vi "Read Tektronix Configuration.vi"(8 "error in (no error)":errorcluster, 11 "Tektronix Driver in":refnum<class "Tektronix Driver.lvclass">) -> (0 "error out":errorcluster, 2 "Tektronix Configuration":T1={"Channel"=0, "Number of averages"=4096, "Input Impedance"=0, "Timebase"=1e-06, "Input range"=2.0} {"Input range" format="%#_6pV"; "Timebase" format="%#_6ps"; "Input Impedance" items=["1M", "50", "Isolated"]}, 3 "Tektronix Driver out":refnum<class "Tektronix Driver.lvclass">)   [LabVIEW 2021, in "Tektronix Driver.lvclass"]
uses:
  Tektronix Driver.lvclass
  Tektronix Configuration.ctl
  Tektronix Driver.lvclass/Tektronix Driver.ctl
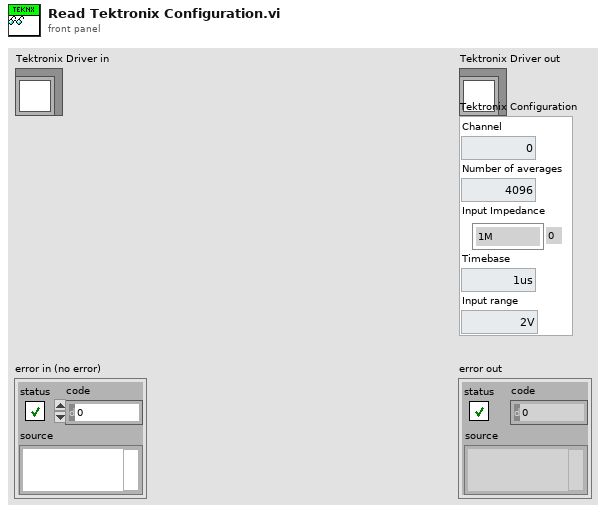
[diagram p1: front panel]
types:
  T1 = typedef "Tektronix Configuration.ctl" = cluster{"Channel":i32, "Number of averages":i32, "Input Impedance":u16, "Timebase":dbl, "Input range":dbl}
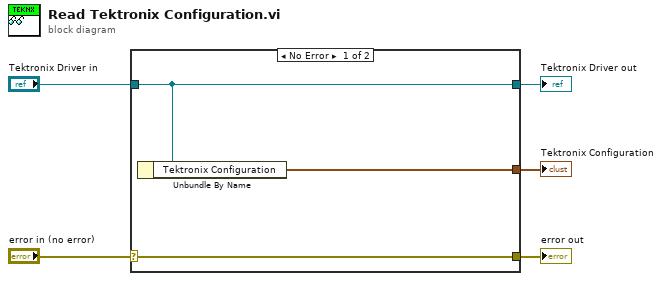
[diagram p0: block diagram]
diagram:
  n1 = case shown="No Error" "error in (no error)" {
    selector: "error in (no error)" -> [w8 w9]
    tunnel: [w8 w9] -> w4
    tunnel: [w7 w10] -> w2
    tunnel: "Tektronix Driver in" -> [w7 w10]
    tunnel: [w6 _] -> w1
    frame No Error {
      n2 = Unbundle By Name(w7) -> ("Tektronix Configuration"=w6:T1)
    }
    frame Error {
    }
  }
  "error out" <- w4
  "Tektronix Driver out" <- w2
  "Tektronix Configuration" <- w1
